vi "Top segment value_test2.vi"(10 "Top player segment position":string) -> (1 "Top player segment value":i32, 2 "Top player court segment display":bool[][](array[boolean]))   [LabVIEW 2013]
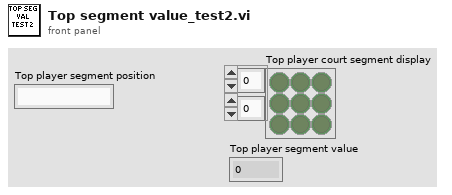
[diagram p1: front panel]
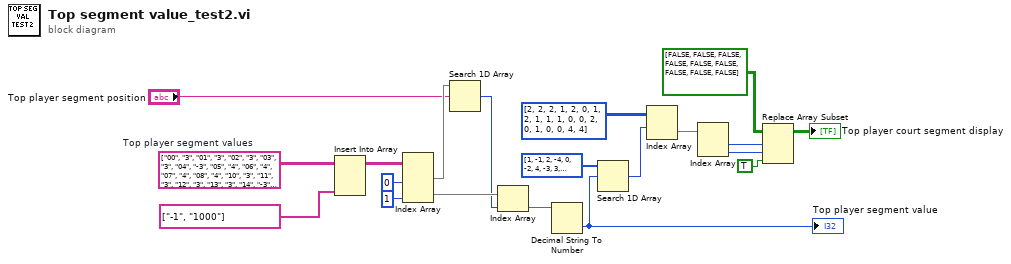
[diagram p0: block diagram]
diagram:
  w12 = string[][] [["00", "3"], ["01", "3"], ["02", "3"], ["03", "3"], ["04", "-3"], ["05", "4"], ["06", "4"], ["07", "4"], ["08", "4"], ["10", "3"], ["11", "3"], ["12", "3"], ["13", "3"], ["14", "-3"], ["15", "4"], ["16", "4"], ["17", "4"], ["18", "4"], ["20", "3"], ["21", "3"], ["22", "3"], ["23", "3"], ["24", "-3"], ["25", "4"], ["26", "4"], ["27", "4"], ["28", "4"], ["30", "3"], ["31", "3"], ["32", "3"], ["33", "0"], ["34", "0"], ["35", "0"], ["36", "4"], ["37", "4"], ["38", "4"], ["40", "-2"], ["41", "-2"], ["42", "-2"], ["43", "0"], ["44", "0"], ["45", "0"], ["46", "-4"], ["47", "-4"], ["48", "-4"], ["50", "2"], ["51", "2"], ["52", "2"], ["53", "0"], ["54", "0"], ["55", "0"], ["56", "1"], ["57", "1"], ["58", "1"], ["60", "2"], ["61", "2"], ["62", "2"], ["63", "2"], ["64", "-1"], ["65", "1"], ["66", "1"], ["67", "1"], ["68", "1"], ["70", "2"], ["71", "2"], ["72", "2"], ["73", "2"], ["74", "-1"], ["75", "1"], ["76", "1"], ["77", "1"], ["78", "1"], ["80", "2"], ["81", "2"], ["82", "2"], ["83", "2"], ["84", "-1"], ["85", "1"], ["86", "1"], ["87", "1"], ["88", "1"]]  # Top player segment values
  n1 = Insert Into Array(array=w12, new element=string[] ["-1", "1000"] ("new element/subarray")) -> (w11:string[][])  [unwired: 2 in]
  n2 = Index Array(array=w11, index (col) #1=0 ("disabled index (col)"), index (col) #2=1 ("index (col)")) -> (element #1=w19:string[], element #2=w16:string[])  [unwired: 2 in]
  n3 = Search 1D Array(1D array=w19, element="Top player segment position") -> (index of element=w15:i32)  [unwired: 1 in]
  n4 = Index Array(array=w16, index=w15) -> (element=w14:string)
  n5 = Decimal String To Number(string=w14) -> (number=w9:i32)  [unwired: 2 in, 1 out]
  "Top player segment value" <- w9
  n6 = Search 1D Array(1D array=i32[] [1, -1, 2, -4, 0, -2, 4, -3, 3, 1000], element=w9) -> (index of element=w7:i32)  [unwired: 1 in]
  n7 = Index Array(array=i32[][] [[2, 2], [2, 1], [2, 0], [1, 2], [1, 1], [1, 0], [0, 2], [0, 1], [0, 0], [4, 4]], index (row)=w7) -> (element=w6:i32[])  [unwired: 1 in]
  n8 = Index Array(array=w6) -> (element #1=w4:i32, element #2=w3:i32)  [unwired: 2 in]
  n9 = Replace Array Subset(array=bool[][] [[FALSE, FALSE, FALSE], [FALSE, FALSE, FALSE], [FALSE, FALSE, FALSE]] ("Top player court segment display"), new element=TRUE ("new element/subarray"), index (row)=w4, index (col)=w3) -> (→"Top player court segment display":bool[][])
